vi "Globals.vi"() -> ()   [LabVIEW 2019, in "ACSVcontrol-driver.lvlib"]
doc: "Globals of the driver storing IP addres, timeouts, abort and status refnum"
uses:
  ACSVcontrol-driver.lvlib
  Public/Type Definitions/Timeouts.ctl
  Public/Type Definitions/Debug status.ctl
  Type definitions/Debug data.ctl
panel:
  in  "Simulation mode":bool
  out "Debug data array":T1[](array[typedef]) {"Time Stamp" format="%<%.3X %x>T"}
  in  "Debug mode":T2=enum."Off"
  in  "Abort Refnum":refnum<vi>
  in  "Status Refnum":refnum<vi>
  in  "IP address:port":string="192.168.1.2:31180"
  in  "Timeouts":T3={"TCP Read & Write (ms)"=7000, "Sensors readout"=5000, "PJVS setup"=10000, "Nullmeter readout"=5000, "Multiplexer setup"=3000, "57XX setup"=5000, "Generator setup"=5000, "Synthesizer setup"=3000, "Sampler readout"=10000}
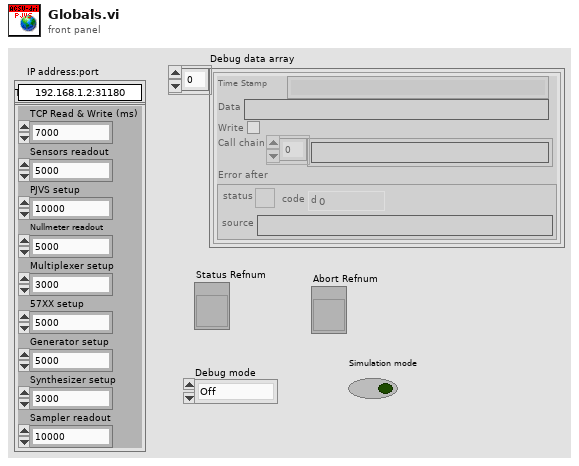
[diagram p1: front panel]
types:
  T1 = typedef "ACSVcontrol-driver.lvlib/Debug data.ctl" = cluster{"Time Stamp":timestamp, "Data":string, "Write":bool, "Call chain":string[], "Error after":errorcluster}
  T2 = typedef "ACSVcontrol-driver.lvlib/Debug status.ctl" = enum16{"No change", "Off", "On"}
  T3 = typedef "ACSVcontrol-driver.lvlib/Timeouts.ctl" = cluster{"TCP Read & Write (ms)":i32, "Sensors readout":i32, "PJVS setup":i32, "Nullmeter readout":i32, "Multiplexer setup":i32, "57XX setup":i32, "Generator setup":i32, "Synthesizer setup":i32, "Sampler readout":i32}
diagram:
